vi "Box_Boundary.vi"(8 "error in":errorcluster, 10 "Boundary":T2={"X max"=310.0, "X min"=147.0, "Z max"=148.0, "Z min"=-92.0}, 11 "Calibrated Oculus Data":T1) -> (0 "error out":errorcluster, 3 "Calibrated Oculus Data 2":T1)   [LabVIEW 2017]
uses:
  Calibrated Oculus Data.ctl
  <vilib>/express/express arith-compare/Formula/XNode/ExpressFormulaBlockNode.xnode
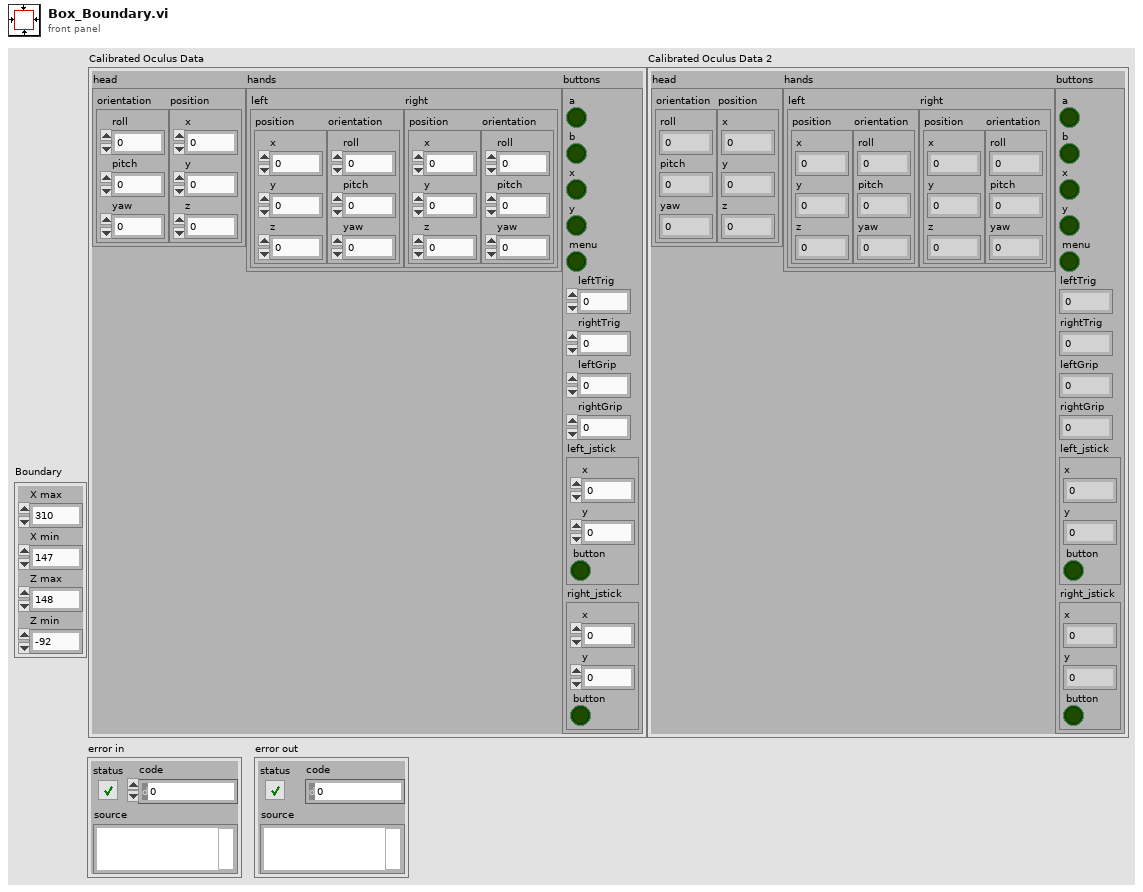
[diagram p1: front panel]
types:
  T1 = typedef "Calibrated Oculus Data.ctl" = cluster{"head":cluster{"orientation":cluster{"roll":dbl, "pitch":dbl, "yaw":dbl}, "position":cluster{"x":dbl, "y":dbl, "z":dbl}}, "hands":cluster{"left":cluster{"position":cluster{"x":dbl, "y":dbl, "z":dbl}, "orientation":cluster{"roll":dbl, "pitch":dbl, "yaw":dbl}}, "right":cluster{"position":cluster{"x":dbl, "y":dbl, "z":dbl}, "orientation":cluster{"roll":dbl, "pitch":dbl, "yaw":dbl}}}, "buttons":cluster{"a":bool, "b":bool, "x":bool, "y":bool, "menu":bool, "leftTrig":dbl, "rightTrig":dbl, "leftGrip":dbl, "rightGrip":dbl, "left_jstick":cluster{"x":dbl, "y":dbl, "button":bool}, "right_jstick":cluster{"x":dbl, "y":dbl, "button":bool}}}
  T2 = cluster{"X max":dbl, "X min":dbl, "Z max":dbl, "Z min":dbl}
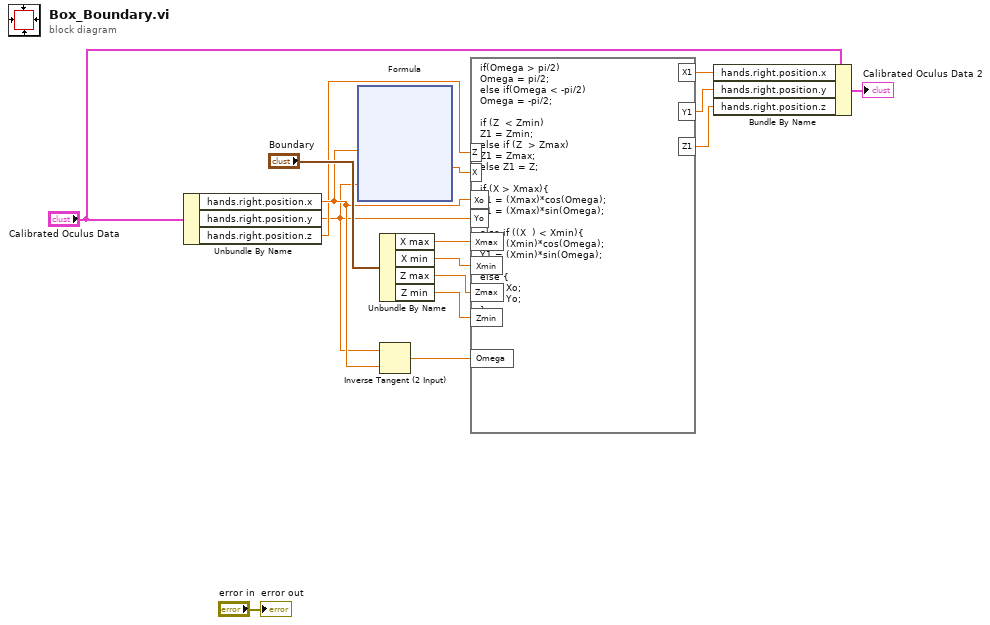
[diagram p0: block diagram]
diagram:
  n1 = Unbundle By Name("Calibrated Oculus Data") -> ("hands.right.position.x"=w9:dbl, "hands.right.position.y"=w4:dbl, "hands.right.position.z"=w5:dbl)
  n2 = xnode "Formula"("Xo"=w9, "Yo"=w4) -> ("Result"=w11:dbl)  [unwired: 1 in, 1 out]
  n3 = Unbundle By Name("Boundary") -> ("X max"=w15:dbl, "X min"=w14:dbl, "Z max"=w12:dbl, "Z min"=w13:dbl)
  n4 = Inverse Tangent (2 Input)(1:w9, 2:w4) -> (0:w10:dbl)
  n5 = formula code="if(Omega > pi/2)\nOmega = pi/2;\nelse if(Omega < -pi/2)\nOmega = -pi/2;\n\nif (Z  < Zmin)\nZ1 = Zmin;\nelse if (Z  > Zmax)\nZ1 = Zmax;\nelse Z1 = Z;\n\nif (X > Xmax){\nX1 = (Xmax)*cos(Omega);\nY1 = (Xmax)*sin(Omega);\n}\nelse if ((X  ) < Xmin){\nX1 = (Xmin)*cos(Omega);\nY1 = (Xmin)*sin(Omega);\n}\nelse {\nX1 = Xo;\nY1 = Yo;\n}"("X"=w11, "Z"=w5, "Zmin"=w13, "Zmax"=w12, "Xmin"=w14, "Xmax"=w15, "Omega"=w10, "Xo"=w9, "Yo"=w4) -> ("Z1"=w6:dbl, "X1"=w8:dbl, "Y1"=w7:dbl)
  n6 = Bundle By Name(cluster="Calibrated Oculus Data", "hands.right.position.x"=w8, "hands.right.position.y"=w7, "hands.right.position.z"=w6) -> (→"Calibrated Oculus Data 2":T1)
  "error out" <- "error in"
